vi "OEE_SCREEN_2_line_bottleneck_into_cluster.vi"(6 "SCREEN_2":T2={"header_part_no"="-", "header_customer"="-", "performance_percentage"="-", "performance_target"="-", "performance_actual"="-", "performance_header"="PERFORMANCE", "performance_header_target"="TARGET", "performance_header_actual"="ACTUAL"}, 11 "SCREEN_1":T1={"header_date"="-", "header_time"="-", "header_takt"="-", "header_shift"="-", "OP10_actual"="-", "OP10_rejects"="-", "OP10_quality_yeild"="-", "OP10_pace"="-", "OP20_actual"="-", "OP20_rejects"="-", "OP20_quality_yeild"="-", "OP20_pace"="-", "OP30_actual"="-", "OP30_rejects"="-", "OP30_quality_yeild"="-", "OP30_pace"="-", "OP40_actual"="-", "OP40_rejects"="-", "OP40_quality_yeild"="-", "OP40_pace"="-", "OP50_actual"="-", "OP50_rejects"="-", "OP50_quality_yeild"="-", "OP50_pace"="-", "OP60_actual"="-", "OP60_rejects"="-", "OP60_quality_yeild"="-", "OP60_pace"="-", "OP70_actual"="-", "OP70_rejects"="-", "OP70_quality_yeild"="-", "OP70_pace"="-", "OP80_actual"="-", "OP80_rejects"="-", "OP80_quality_yeild"="-", "OP80_pace"="-", "OP90_actual"="-", "OP90_rejects"="-", "OP90_quality_yeild"="-", "OP90_pace"="-", "OP100_actual"="-", "OP100_rejects"="-", "OP100_quality_yeild"="-", "OP100_pace"="-", "OP110_actual"="-", "OP110_rejects"="-", "OP110_quality_yeild"="-", "OP110_pace"="-", "OP120_actual"="-", "OP120_rejects"="-", "OP120_quality_yeild"="-", "OP120_pace"="-", "OP130_actual"="-", "OP130_rejects"="-", "OP130_quality_yeild"="-", "OP130_pace"="-", "OP10_header"="OP10", "OP20_header"="OP20", "OP30_header"="OP30", "OP40_header"="OP40", "OP50_header"="OP50", "OP60_header"="OP60", "OP70_header"="OP70", "OP80_header"="OP80", "OP90_header"="OP90", "OP100_header"="OP100", "OP110_header"="OP110", "OP120_header"="OP120", "OP130_header"="OP130", "additional_info"="", "bottleneck_OP"="-", "bottleneck_header"="LINE BOTTLENECK"}) -> (4 "SCREEN_2":T2={"header_part_no"="-", "header_customer"="-", "performance_percentage"="-", "performance_target"="-", "performance_actual"="-", "performance_header"="PERFORMANCE", "performance_header_target"="TARGET", "performance_header_actual"="ACTUAL"})   [LabVIEW 2019]
uses:
  FGV/SQL_raw_data/FGV_OEE_SQL_raw_data.ctl
  typedef/SCREEN_2.ctl
  SCREEN_1/typedef/SCREEN_1.ctl
panel:
  # "PERFORMANCE DATA OUTPUT BOARD #1"
  # "OP"
  # "Actual"
  # "Rejects"
  # "%FTTH"
  # "Pace"
  # "OP"
  # "Actual"
  # "Rejects"
  # "%FTTH"
  # "Pace"
  # "Performance Data Output Board #2"
  # "Performance Data Output Board #2"
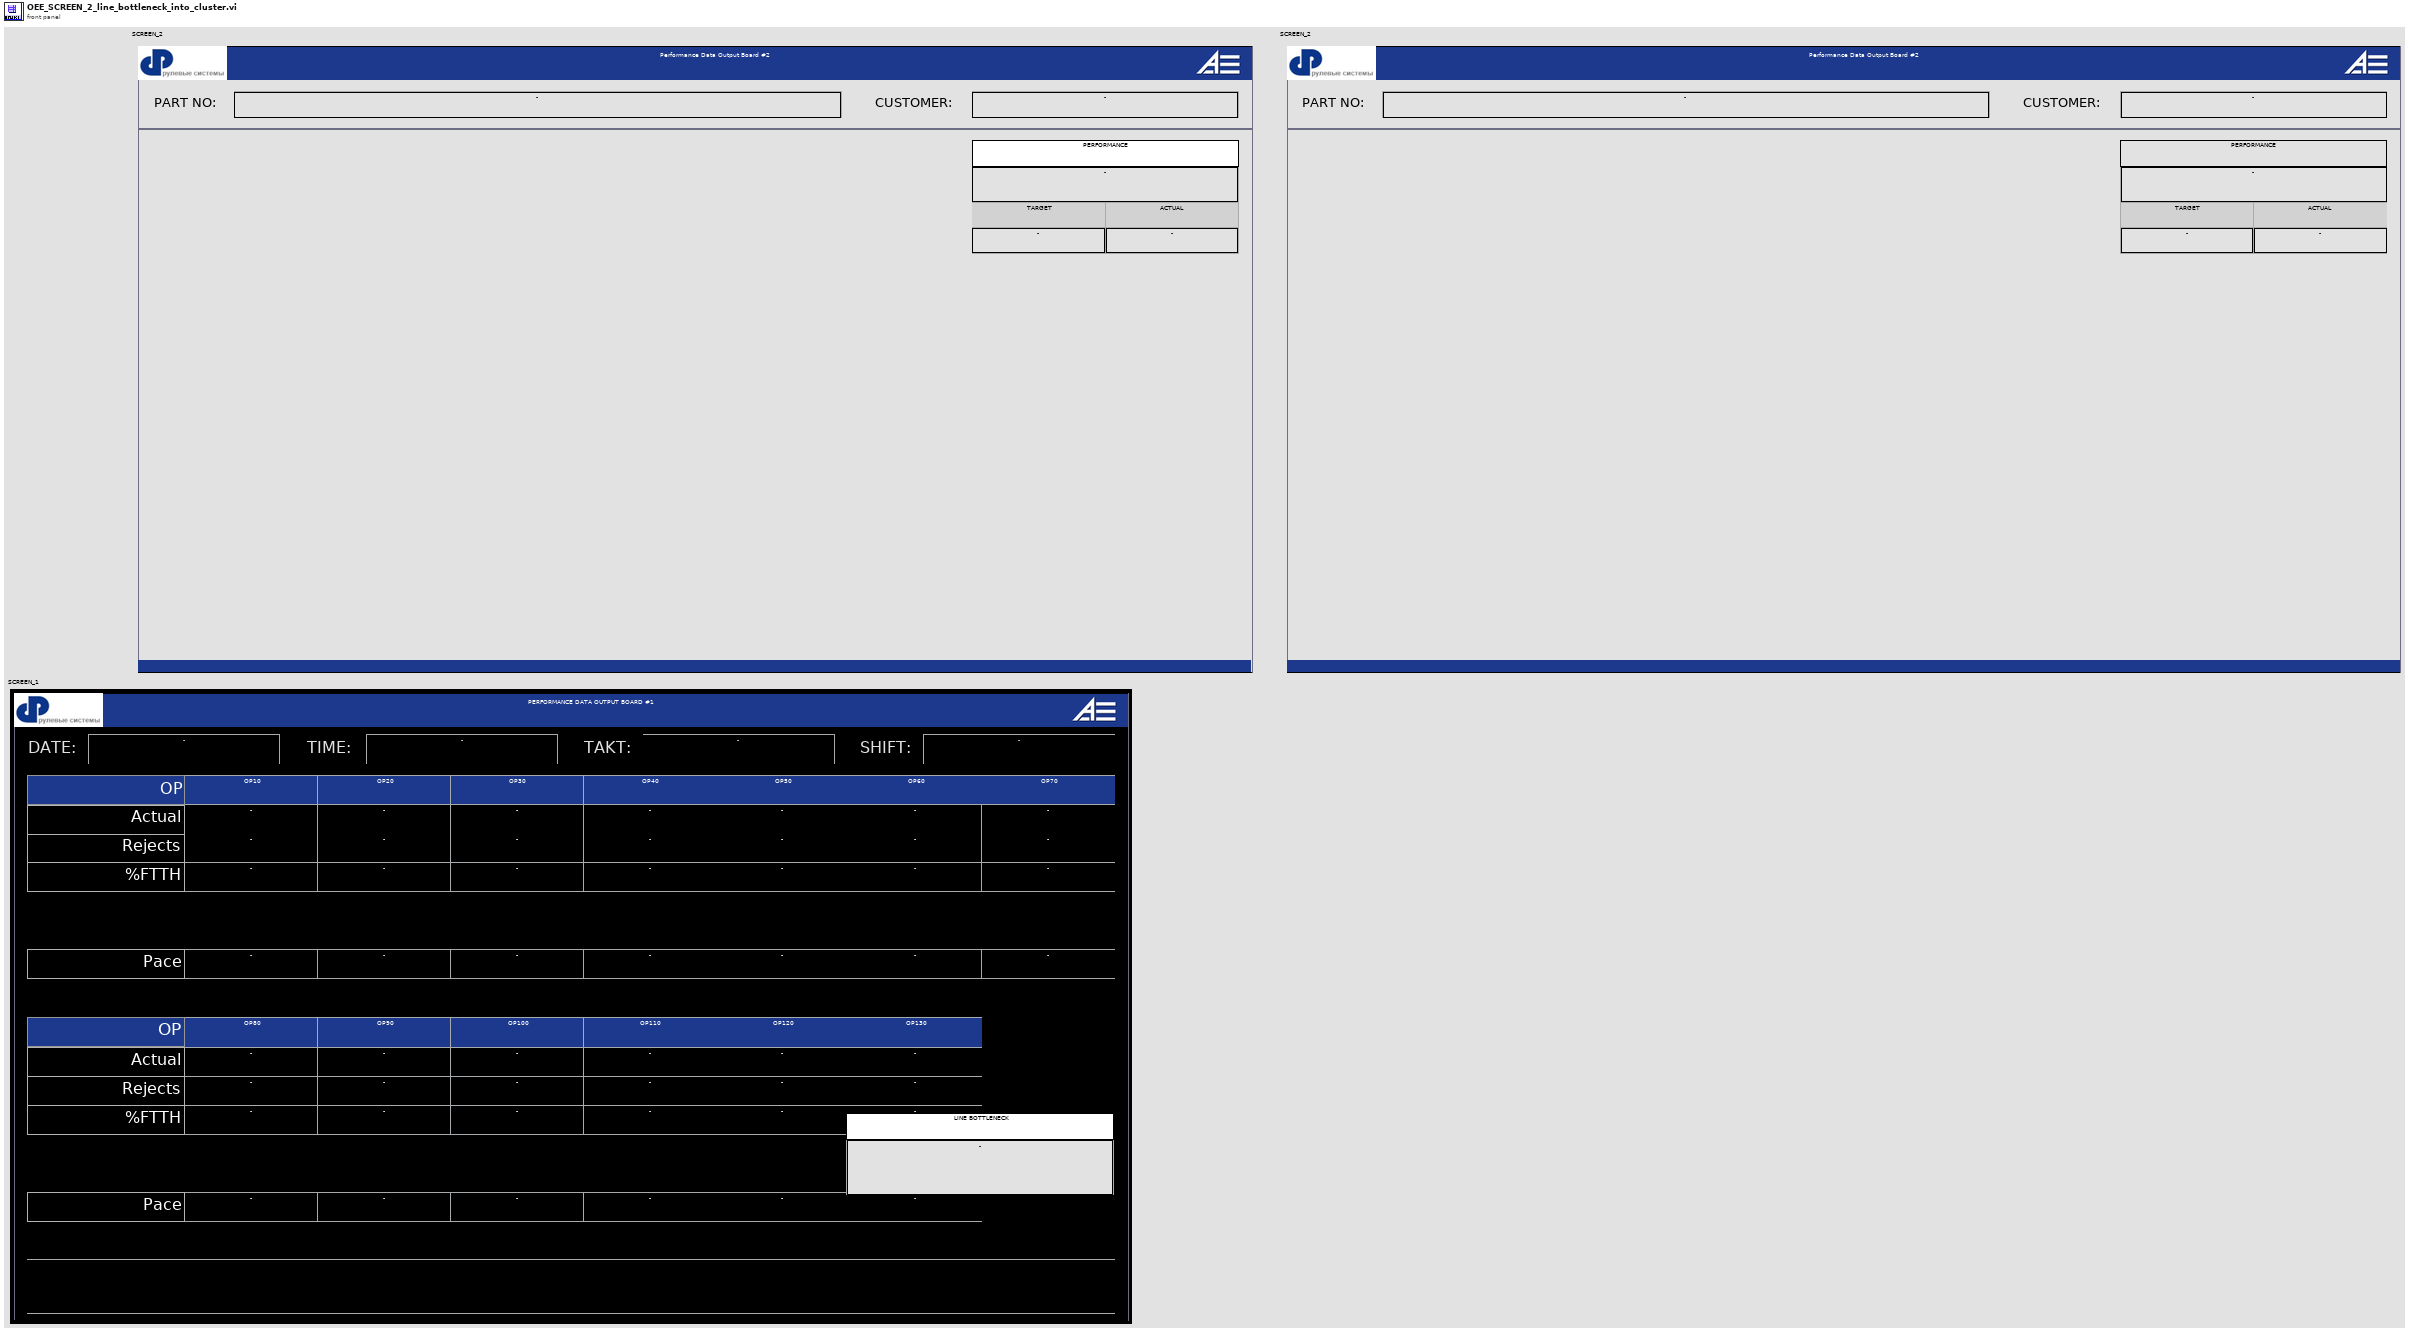
[diagram p1: front panel]
types:
  T1 = typedef "SCREEN_1.ctl" = cluster{"header_date":string, "header_time":string, "header_takt":string, "header_shift":string, "OP10_actual":string, "OP10_rejects":string, "OP10_quality_yeild":string, "OP10_pace":string, "OP20_actual":string, "OP20_rejects":string, "OP20_quality_yeild":string, "OP20_pace":string, "OP30_actual":string, "OP30_rejects":string, "OP30_quality_yeild":string, "OP30_pace":string, "OP40_actual":string, "OP40_rejects":string, "OP40_quality_yeild":string, "OP40_pace":string, "OP50_actual":string, "OP50_rejects":string, "OP50_quality_yeild":string, "OP50_pace":string, "OP60_actual":string, "OP60_rejects":string, "OP60_quality_yeild":string, "OP60_pace":string, "OP70_actual":string, "OP70_rejects":string, "OP70_quality_yeild":string, "OP70_pace":string, "OP80_actual":string, "OP80_rejects":string, "OP80_quality_yeild":string, "OP80_pace":string, "OP90_actual":string, "OP90_rejects":string, "OP90_quality_yeild":string, "OP90_pace":string, "OP100_actual":string, "OP100_rejects":string, "OP100_quality_yeild":string, "OP100_pace":string, "OP110_actual":string, "OP110_rejects":string, "OP110_quality_yeild":string, "OP110_pace":string, "OP120_actual":string, "OP120_rejects":string, "OP120_quality_yeild":string, "OP120_pace":string, "OP130_actual":string, "OP130_rejects":string, "OP130_quality_yeild":string, "OP130_pace":string, "OP10_header":string, "OP20_header":string, "OP30_header":string, "OP40_header":string, "OP50_header":string, "OP60_header":string, "OP70_header":string, "OP80_header":string, "OP90_header":string, "OP100_header":string, "OP110_header":string, "OP120_header":string, "OP130_header":string, "additional_info":string, "bottleneck_OP":string, "bottleneck_header":string}
  T2 = typedef "SCREEN_2.ctl" = cluster{"header_part_no":string, "header_customer":string, "performance_percentage":string, "performance_target":string, "performance_actual":string, "performance_header":string, "performance_header_target":string, "performance_header_actual":string}
  T3 = typedef "FGV_OEE_SQL_raw_data.ctl" = enum16{"initialize", "set_reference_name", "set_timestamp", "set_OK_NOK_count", "set_config_info", "set_cycle_time_and_pace", "set_last_operator", "set_availability", "set_hourly_ok_count", "set_targets", "get_all_info"}
  T4 = typedef "OEE_SQL_raw_data.ctl" = cluster{"reference_name":string, "data_timestamp":timestamp, "OK_NOK_count":string[][], "config_info":string[], "pace":string[][], "last_operator":string[][], "availability":string[], "hourly_ok_count":string[][], "shift_start":i8, "shift_end":i8, "TAKT":u16, "FTTH_target":u16, "OEE_target":u16, "BOTTLENECK_station":u16, "targets_hourly":u16[], "target_shift":u16}
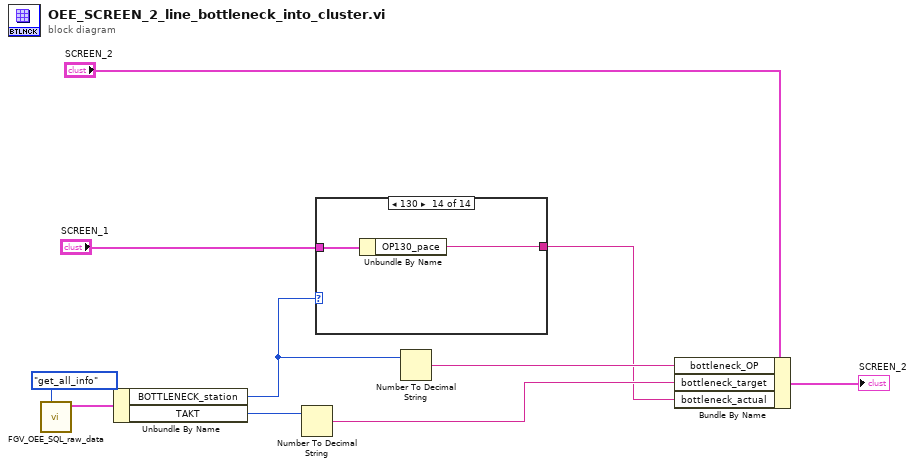
[diagram p0: block diagram]
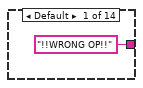
[diagram p2: hidden frame]
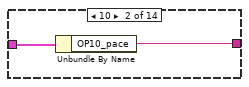
[diagram p3: hidden frame]
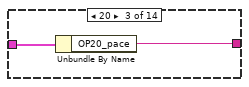
[diagram p4: hidden frame]
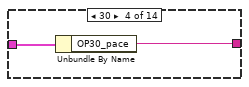
[diagram p5: hidden frame]
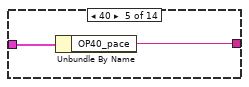
[diagram p6: hidden frame]
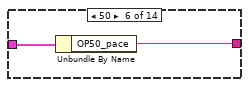
[diagram p7: hidden frame]
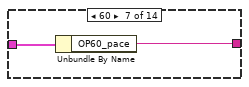
[diagram p8: hidden frame]
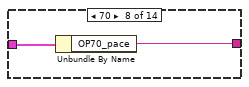
[diagram p9: hidden frame]
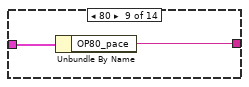
[diagram p10: hidden frame]
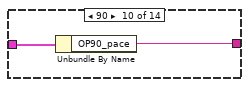
[diagram p11: hidden frame]
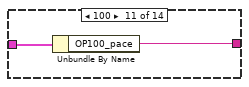
[diagram p12: hidden frame]
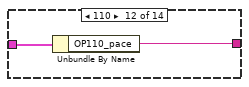
[diagram p13: hidden frame]
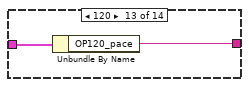
[diagram p14: hidden frame]
diagram:
  n1 = call "FGV_OEE_SQL_raw_data.vi"("options"=FGV_OEE_SQL_raw_data."get_all_info") -> ("SQL_raw_data_out"=w7:T4)  [unwired: 9 in, 1 out]
  n2 = Unbundle By Name(w7) -> ("BOTTLENECK_station"=w3:u16, "TAKT"=w6:u16)
  n3 = Number To Decimal String(number=w6) -> (decimal integer string=w5:string)  [unwired: 1 in]
  n4 = case shown="130" w3 {
    tunnel: "SCREEN_1" -> [_ w13 w15 w17 w19 w21 w23 w25 w27 w29 w31 w33 w35 w37]
    tunnel: ["!!WRONG OP!!" ("OP10_pace") w12 w14 w16 w18 w20 w22 w24 w26 w28 w30 w32 w34 w36] -> w1
    frame Default {
    }
    frame 10 {
      n5 = Unbundle By Name(w13) -> ("OP10_pace"=w12:string)
    }
    frame 20 {
      n6 = Unbundle By Name(w15) -> ("OP20_pace"=w14:string)
    }
    frame 30 {
      n7 = Unbundle By Name(w17) -> ("OP30_pace"=w16:string)
    }
    frame 40 {
      n8 = Unbundle By Name(w19) -> ("OP40_pace"=w18:string)
    }
    frame 50 {
      n9 = Unbundle By Name(w21) -> ("OP50_pace"=w20:string)
    }
    frame 60 {
      n10 = Unbundle By Name(w23) -> ("OP60_pace"=w22:string)
    }
    frame 70 {
      n11 = Unbundle By Name(w25) -> ("OP70_pace"=w24:string)
    }
    frame 80 {
      n12 = Unbundle By Name(w27) -> ("OP80_pace"=w26:string)
    }
    frame 90 {
      n13 = Unbundle By Name(w29) -> ("OP90_pace"=w28:string)
    }
    frame 100 {
      n14 = Unbundle By Name(w31) -> ("OP100_pace"=w30:string)
    }
    frame 110 {
      n15 = Unbundle By Name(w33) -> ("OP110_pace"=w32:string)
    }
    frame 120 {
      n16 = Unbundle By Name(w35) -> ("OP120_pace"=w34:string)
    }
    frame 130 {
      n17 = Unbundle By Name(w37) -> ("OP130_pace"=w36:string)
    }
  }
  n18 = Number To Decimal String(number=w3) -> (decimal integer string=w4:string)  [unwired: 1 in]
  n19 = Bundle By Name(cluster="SCREEN_2", "bottleneck_OP"=w4, "bottleneck_target"=w5, "bottleneck_actual"=w1) -> (→"SCREEN_2":T2)
